vi "circular_fitting(subVI).vi"(7 "Color":u32(colorbox)=16711680, 8 "error in (no error)":errorcluster, 11 "Image":T5=refnum) -> (0 "error out":errorcluster, 2 "Image Out":T5, 3 "Circle out":T6 {"Radius" format="%.2f"; "Center"."Y" format="%.2f"; "Center"."X" format="%.2f"}, 5 "Circle Found":bool)   [LabVIEW 2020]
uses:
  <vilib>/vision/Image Controls.llb/IMAQ Image.ctl
  <vilib>/vision/Measure.llb/Edge Options.ctl
  <vilib>/vision/Measure.llb/Edge Polarity.ctl
  <vilib>/vision/NI_Vision_Development_Module.lvlib
panel:
  in  "Options":T3={"Search  Direction"=0, "Edge Options"={"Edge Polarity"=0, "Kernel Size"=3, "Width"=3, "Minimum Edge Strength"=10.0, "Interpolation Type"=enum."Bilinear Fixed", "Data Processing Method"=enum."Average"}, "Show Search Area"=FALSE, "Show Search Lines"=FALSE, "Show Edges Found"=FALSE, "Show Result"=TRUE, "Search Area Color"=65280, "Search Lines Color"=255, "Edge Locations Color"=16776960, "Result Color"=16711680, "Overlay Group Name"=""} {"Search  Direction" items=["Outside to Inside", "Inside to Outside"]; "Edge Options"."Edge Polarity" items=["All Edges", "Rising Edges", "Falling Edges"]; "Edge Options"."Minimum Edge Strength" format="%.2f"; "Edge Options"."Width" step=2; "Edge Options"."Kernel Size" step=2}
  in  "Circle Fit Options":T4={"Process"=enum."Get Best Edge", "Step Size"=3.0, "Max Pixel Radius"=1000}
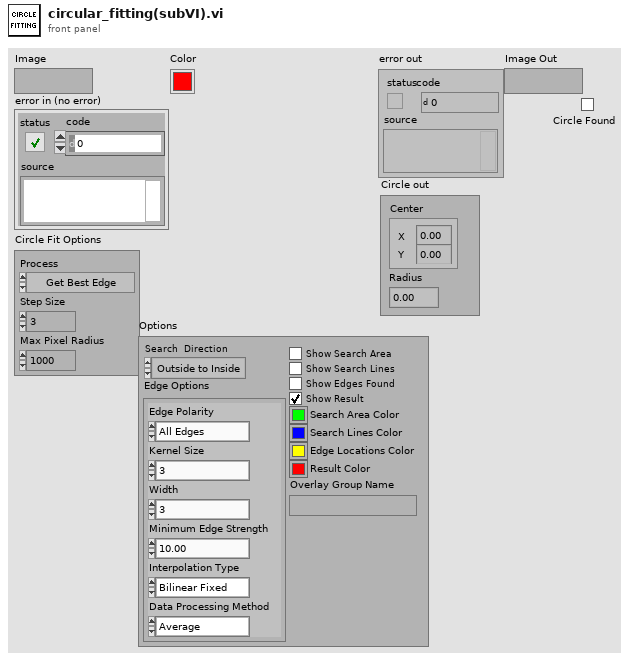
[diagram p1: front panel]
types:
  T1 = typedef "Edge Options.ctl" = cluster{"Edge Polarity":T2, "Kernel Size":u32, "Width":u32, "Minimum Edge Strength":sgl, "Interpolation Type":enum32{"Zero Order", "Bilinear", "Quadratic", "Cubic", "Bilinear Fixed"}, "Data Processing Method":enum32{"Average", "Median"}}
  T2 = typedef "Edge Polarity.ctl" = u32
  T3 = cluster{"Search  Direction":u32, "Edge Options":T1, "Show Search Area":bool, "Show Search Lines":bool, "Show Edges Found":bool, "Show Result":bool, "Search Area Color":u32, "Search Lines Color":u32, "Edge Locations Color":u32, "Result Color":u32, "Overlay Group Name":string}
  T4 = cluster{"Process":enum16{"Get First Edge", "Get First + Last Edge", "Get All Edges", "Get Best Edge"}, "Step Size":dbl, "Max Pixel Radius":i32}
  T5 = typedef "IMAQ Image.ctl" = refnum<image>
  T6 = cluster{"Center":cluster{"X":sgl, "Y":sgl}, "Radius":dbl}
  T7 = typedef "ROI Descriptor" = cluster{"Global Rectangle":i32[], "Contours":cluster{"ID":enum32{"External", "Internal"}, "Type":u32, "Coordinates":i32[]}[]}
  T8 = cluster{"Center (Pixels)":cluster{"X":sgl, "Y":sgl}, "Radius (Pixels)":dbl, "Center (Real-World)":cluster{"X":sgl, "Y":sgl}, "Radius (Real-World)":dbl, "Roundness (Real-World)":dbl, "Average Strength":dbl, "Average SNR (dB)":dbl}
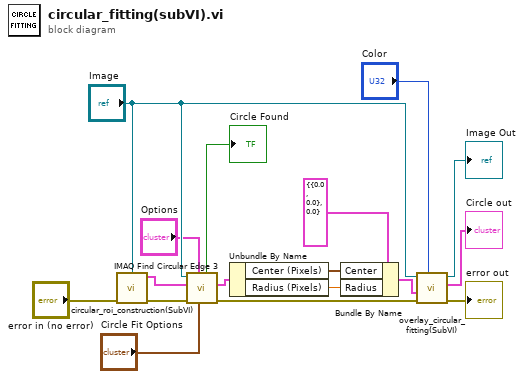
[diagram p0: block diagram]
diagram:
  n1 = call "circular_roi_construction(SubVI).vi"("error in (no error)"="error in (no error)", "image in"="Image") -> ("error out"=w17:errorcluster, "ROI Descriptor"=w3:T7)  [unwired: 8 in]
  n2 = call "IMAQ Find Circular Edge 3"("Circle Fit Options"="Circle Fit Options", "Options"="Options", "error in (no error)"=w17, "ROI Descriptor"=w3, "Image"="Image") -> ("error out"=w10:errorcluster, "Fitted Circle"=w15:T8, "Circle Found"=→"Circle Found":bool)  [unwired: 2 in, 2 out]
  n3 = Unbundle By Name(w15) -> ("Center (Pixels)"=w13:cluster{"X":sgl, "Y":sgl}, "Radius (Pixels)"=w12:dbl)
  n4 = Bundle By Name(cluster=T6 {"Center"={"X"=0.0, "Y"=0.0}, "Radius"=0.0} ("circle in"), "Center"=w13, "Radius"=w12) -> (w11:T6)
  n5 = call "overlay_circular_fitting(SubVI).vi"("Color"="Color", "error in (no error)"=w10, "circle in"=w11, "image dest"="Image") -> ("error out"=→"error out":errorcluster, "Circle out"=→"Circle out":T6, "Image Out"=→"Image Out":T5)  [unwired: 5 in]
